vi "Helper SubVI - Set Show.vi"(6 "view 5":bool=TRUE, 7 "view 4":bool=TRUE, 8 "view 3":bool=TRUE, 9 "view 2":bool=TRUE, 10 "view":bool=TRUE, 11 "in":cluster{"f0":dbl, "df":dbl, "S(f)":dbl[]}[](array[cluster])) -> (3 "out":cluster{"f0":dbl, "df":dbl, "S(f)":dbl[]}[](array[cluster]))   [LabVIEW 2023]
doc: "Sets the plots."
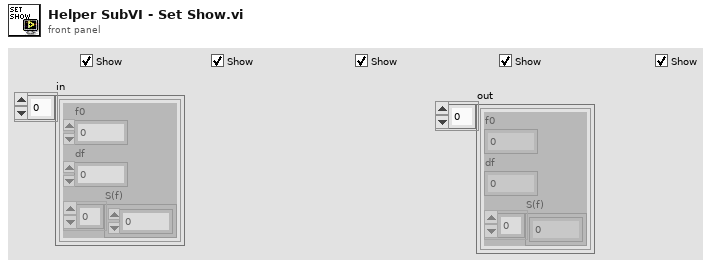
[diagram p1: front panel]
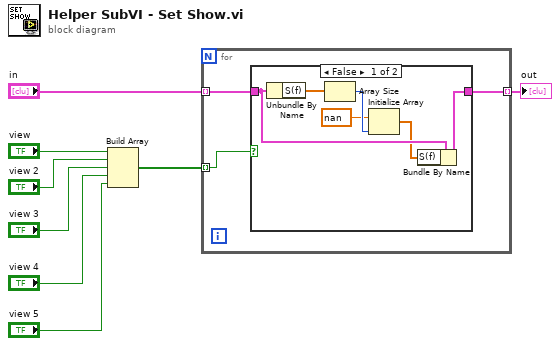
[diagram p0: block diagram]
diagram:
  n1 = Build Array("view", "view 2", "view 3", "view 4", "view 5") -> (w2:bool[])
  n2 = for {
    tunnel: "in" -> [w10] mode=indexing
    tunnel: w2 -> [w11] mode=indexing
    tunnel: [w9] -> w1 mode=indexing
    n3 = case shown="False" w11 {
      tunnel: w10 -> [w14 w18]
      tunnel: [w12 w18] -> w9
      frame False {
        n4 = Unbundle By Name(w14) -> ("S(f)"=w17:dbl[])
        n5 = Array Size(array=w17) -> (size(s)=w16:i32)
        n6 = Initialize Array(nan, w16) -> (w13:dbl[])
        n7 = Bundle By Name(cluster=w14, "S(f)"=w13) -> (w12:cluster{"f0":dbl, "df":dbl, "S(f)":dbl[]})
      }
      frame True {
      }
    }
  }
  "out" <- w1
